vi "ziExample-Module-Impedance.vi"() -> ()   [LabVIEW 2009]
doc: "Control a Zurich instrument device via the LabOne Labview API. \nRequirements: Zurich Instruments MFLI+IA/ MFIA\nThis example shows how to use retrieve impedance data and utilize the sweeper.\n\n© Zurich Instruments AG, www.zhinst.com"
uses:
  <instrlib>/Zurich Instruments LabOne/Public/Modules/ziTypeModSweeperImpedanceWave.ctl
  <instrlib>/Zurich Instruments LabOne/Public/Modules/ziTypeModEnum.ctl
  <instrlib>/Zurich Instruments LabOne/Public/Configure/ziSetValueDoubleArray.vi
  <instrlib>/Zurich Instruments LabOne/Public/Modules/ziModSetValueDoubleArray.vi
  <instrlib>/Zurich Instruments LabOne/Public/Modules/ziModSetValueBinaryArray.vi
  <instrlib>/Zurich Instruments LabOne/Public/Modules/ziModGetSweeperData.vi
  <instrlib>/Zurich Instruments LabOne/Public/Data/ziGetEventImpSample.vi
  <instrlib>/Zurich Instruments LabOne/Public/Configure/ziSetValueDouble.vi
  <instrlib>/Zurich Instruments LabOne/Public/Configure/ziGetValueDouble.vi
  <instrlib>/Zurich Instruments LabOne/Zurich Instruments LabOne.lvlib
  <vilib>/gmath/NI_Gmath.lvlib
panel:
  out "Frequency":dbl
  in  "auto/inputrange":bool caption="Auto"
  in  "voltage/range":dbl=1.0 caption="Range Voltage"
  in  "current/range":dbl=0.001 caption="Range Current"
  in  "output/amplitude":dbl=0.1 caption="Test Signal (V)"
  in  "auto/output":bool caption="Auto"
  in  "model":u16(ring)=1 caption="Model" items=["Rp || Cp", "Rs + Cs", "Rs + Ls", "G B", "D Cs", "Q Cs", "D Ls", "Q Ls", "Rp || Lp", "D Cp"]
  out "?":dbl(graph)
  out "?":dbl(graph)
  in  "Sweep":bool
  in  "Step":dbl=100.0
  in  "stopfreq":dbl=100000.0 caption="Stop Freq"
  in  "startfreq":dbl=1000.0 caption="Start Freq"
  out "Flags":bool[][](array[boolean])
  out "ImpedanceSweeperData":T1 {"bandwidthMode" format="%f"; "flags" format="%f"; "sampleFormat" format="%f"; "sweepMode" format="%f"; "sampleCount" format="%f"; "timestamp" format="%f"}
  in  "stop":bool
  out "IA Parameter 2":dbl
  out "IA Parameter 1":dbl format="%#_6p"
  out "Error Out":errorcluster
  in  "Address":string="DEV"
  out "Selected Device":string
  in  "subscribepath":string="imps/0/sample" caption="Subscribe Path"
  out "Param1":cluster{"grid":dbl[], "r_avg":dbl[]}(graph)
  out "Param 0":cluster{"grid":dbl[], "r_avg":dbl[]}(graph)
  # "ziExample-IMPModul.vi\nRequirements: MFLI + IA / MFIA\nsee block diagram for VI description"
  # "Tested Devices:\n\n- MFLI"
  # "VALID_INTERNAL\nVALID_USER\nAUTORANGE_GATING\n\nOVERFLOW_VOLTAGE\nOVERFLOW_CURRENT\nUNDERFLOW_VOLTAGE\nUNDERFLOW_CURRENT\nFREQ_EXACT\nFREQ_INTERPOLATION\nFREQ_EXTRAPOLATION\n\nSUPPRESSION_PARAM0\nSUPPRESSION_PARAM1\nFREQLIMIT_RANGE_VOLTAGE\nFREQLIMIT_RANGE_Current\nSTRONGCOMPENSATION_PARAM0\nSTRONGCOMPENSATION_PARAM1\n\n\nBWC_BIT0\nBWC_BIT1\nBWC_BIT2\nBWC_BIT3\nOPEN_DETECTION"
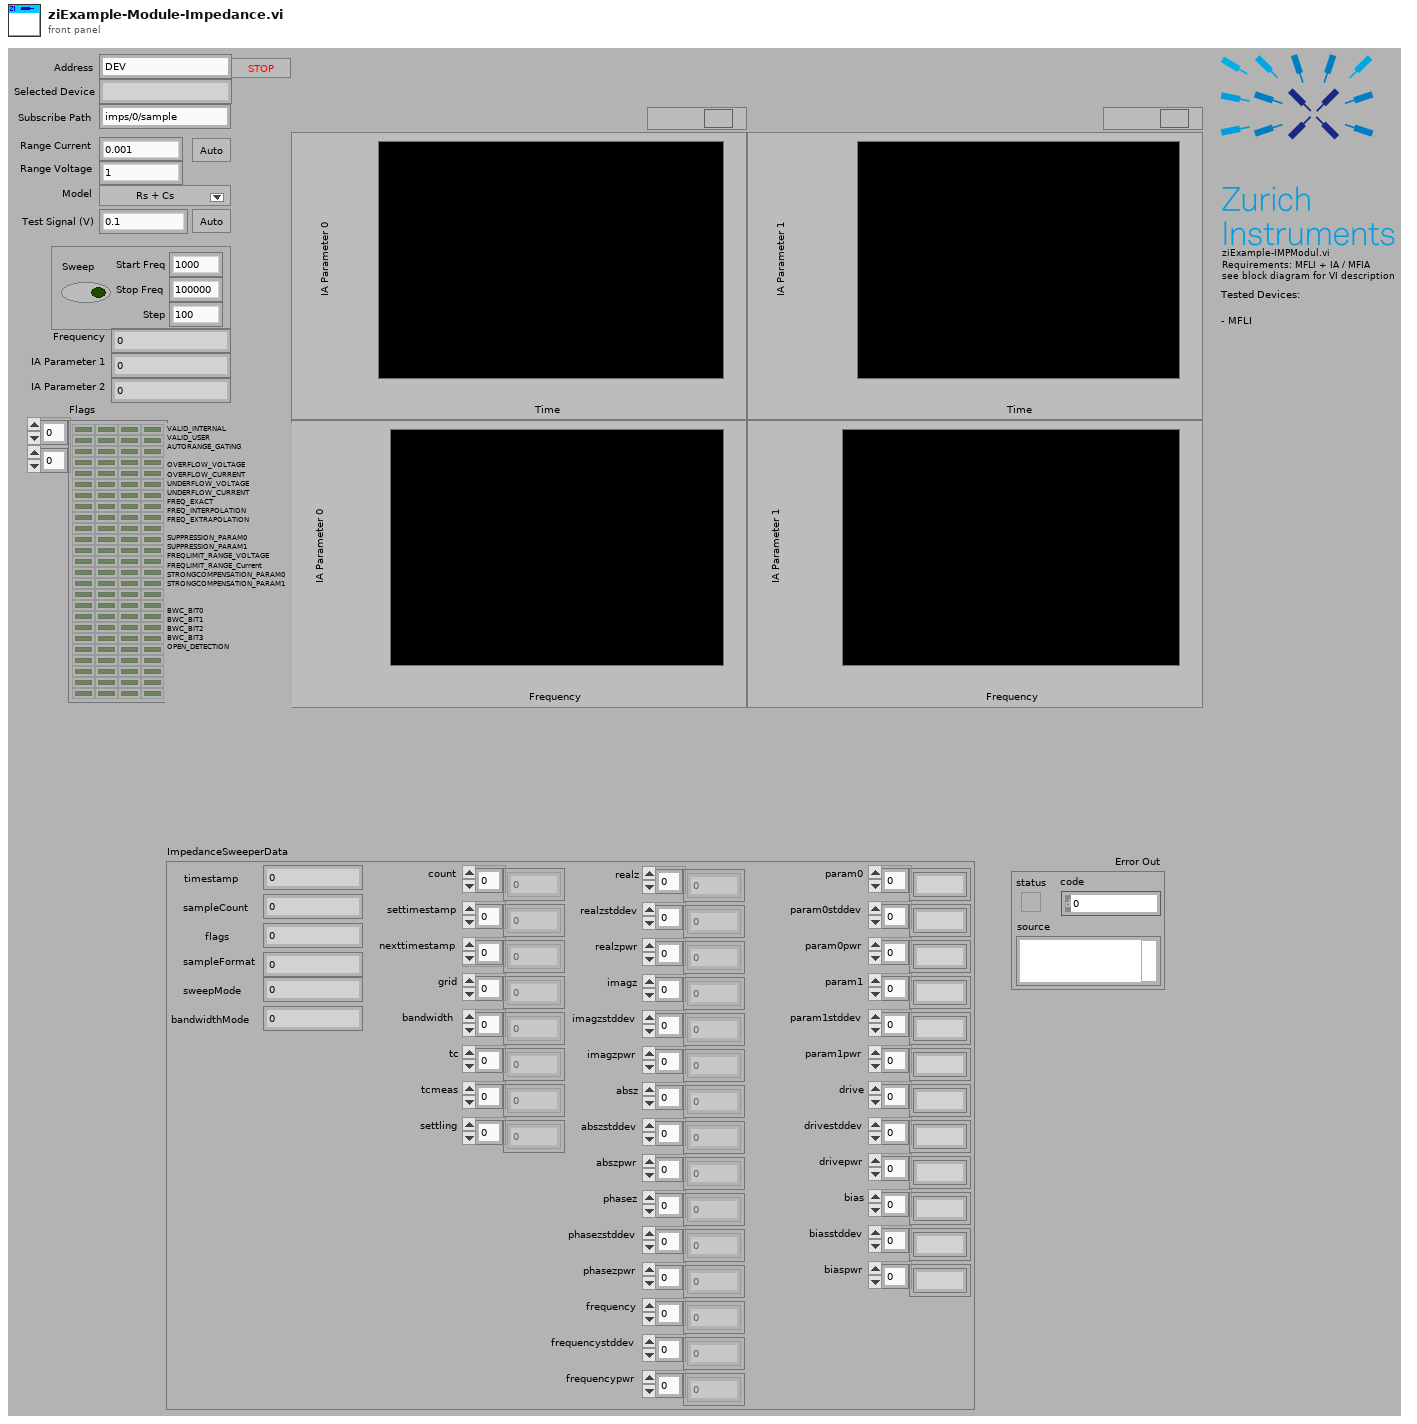
[diagram p1: front panel]
types:
  T1 = typedef "Zurich Instruments LabOne.lvlib/ziTypeModSweeperImpedanceWave.ctl" = cluster{"timestamp":u64, "sampleCount":u64, "flags":u8, "sampleFormat":u8, "sweepMode":u8, "bandwidthMode":u8, "count":u64[], "settimestamp":u64[], "nexttimestamp":u64[], "grid":dbl[], "bandwidth":dbl[], "tc":dbl[], "tcmeas":dbl[], "settling":dbl[], "realz":dbl[], "realzstddev":dbl[], "realzpwr":dbl[], "imagz":dbl[], "imagzstddev":dbl[], "imagzpwr":dbl[], "absz":dbl[], "abszstddev":dbl[], "abszpwr":dbl[], "phasez":dbl[], "phasezstddev":dbl[], "phasezpwr":dbl[], "frequency":dbl[], "frequencystddev":dbl[], "frequencypwr":dbl[], "param0":dbl[], "param0stddev":dbl[], "param0pwr":dbl[], "param1":dbl[], "param1stddev":dbl[], "param1pwr":dbl[], "drive":dbl[], "drivestddev":dbl[], "drivepwr":dbl[], "bias":dbl[], "biasstddev":dbl[], "biaspwr":dbl[]}
  T2 = typedef "Zurich Instruments LabOne.lvlib/ziTypeModEnum.ctl" = u16
  T3 = typedef "Zurich Instruments LabOne.lvlib/ziTypeHandle.ctl" = cluster{"handleValid":bool, "Conn":u64, "Path Prefix":string, "Handle":u64, "Connected":bool, "Clockbase(s)":dbl}
  T4 = typedef "Zurich Instruments LabOne.lvlib/ziTypeModHandle.ctl" = cluster{"handleValid":bool, "Conn":u64, "ModHandle":u64, "moduleID":string, "Path Prefix":string}
  T5 = typedef "Zurich Instruments LabOne.lvlib/ziTypeModResults.ctl" = cluster{"PathArray":string[], "ValueType":T6, "NoOfResults":u64, "ziGenericHeader":T7[]}
  T6 = typedef "Zurich Instruments LabOne.lvlib/ziTypePollType.ctl" = enum16{"NONE", "DOUBLE_DATA", "INTEGER_DATA", "DEMOD_SAMPLE", "SCOPE_WAVE_HF2", "AUXIN_SAMPLE", "DIO_SAMPLE", "BYTE_ARRAY", "PWA_WAVE", "9", "10", "11", "12", "13", "14", "15", "TREE_CHANGE_DEPRI", "17", "ERROR", "19", "20", "21", "22", "23", "24", "25", "26", "27", "28", "29", "30", "31", "DOUBLE_DATA_TS", "INTEGER_DATA_TS", "34", "SCOPE_WAVE", "SCOPE_WAVE_EX", "37", "BYTE_ARRAY_TS", "39", "40", "41", "42", "43", "44", "45", "CNT_DATA", "47", "TREE_CHANGE", "49", "50", "51", "52", "53", "54", "55", "56", "57", "58", "59", "60", "61", "62", "63", "SWEEPER_DATA", "SPECTRUM_DATA", "ADVISOR_DATA", "VECTOR_DATA", "IMP_DATA"}
  T7 = typedef "Zurich Instruments LabOne.lvlib/ziTypeModGenericHeader.ctl" = cluster{"HeaderType":enum8{"HEADER_TYPE_NONE", "HEADER_TYPE_SWTRIGGER", "HEADER_TYPE_SWEEPER"}, "SampleFormat":u8, "SystemTime":timestamp, "CreatedTimeStamp":u64, "ChangedTimeStamp":u64, "Flags":u32, "ChunkSizeBytes":u64, "Name":string, "Status":u32, "GroupIndex":u32, "Color":u32, "ActiveRow":u32, "TriggerNumber":u64, "GridRows":u32, "GridCols":u32, "GridMode":u32, "GridOperation":u32, "GridDirection":u32, "GridRepetitions":u32, "GridColDelta":dbl, "GridColOffset":dbl, "GridRowDelta":dbl, "GridRowOffset":dbl, "Bandwidth":dbl, "Center":dbl, "Nenbw":dbl}
  T8 = typedef "Zurich Instruments LabOne.lvlib/ziTypeImpedanceSample.ctl" = cluster{"Timestamps (ticks)":u64[], "Z (Ohm)":cdb[], "Freq (Hz)":dbl[], "Osc Phase (deg)":dbl[], "Flags":u32[], "Trigger":u32[], "Param0":dbl[], "Param1":dbl[], "Drive":dbl[], "Bias":dbl[]}
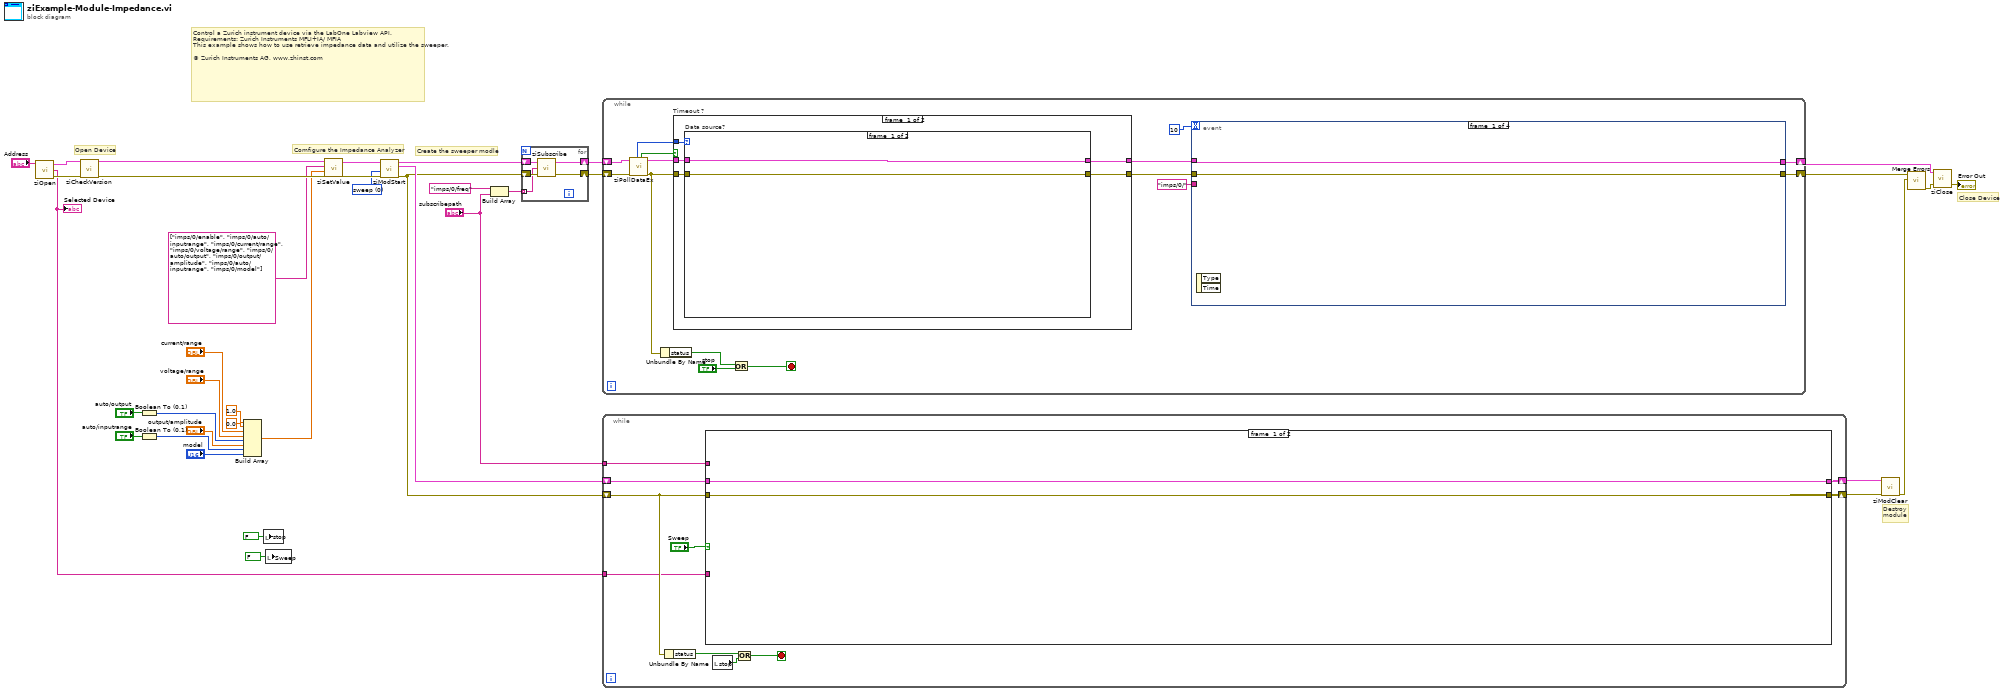
[diagram p0: block diagram]
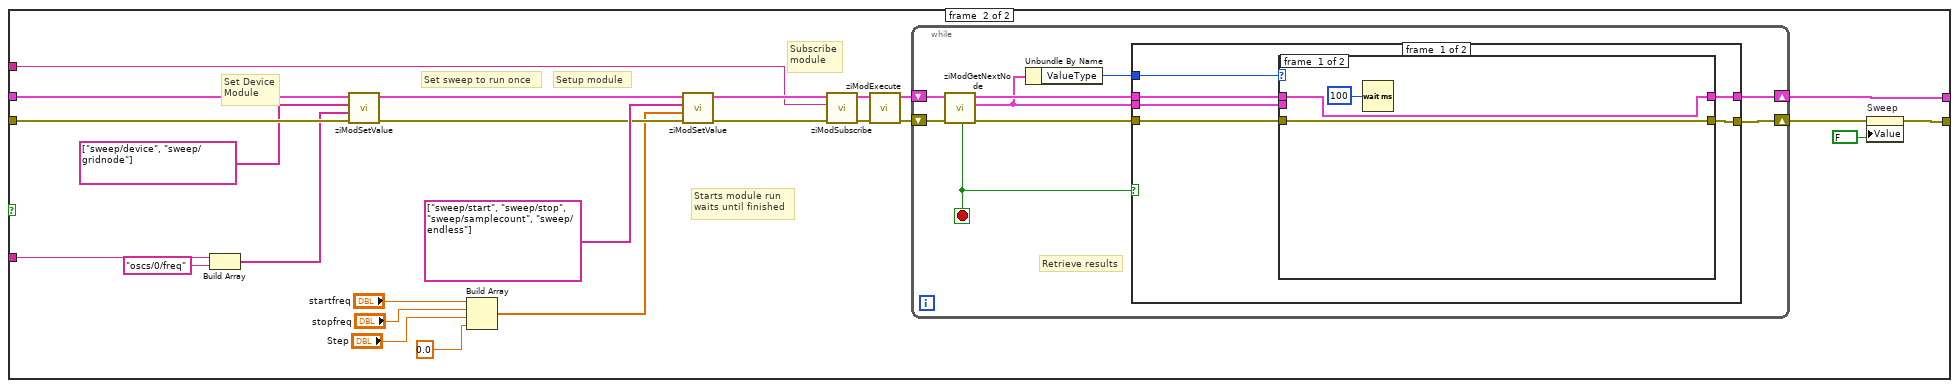
[diagram p2: hidden frame]
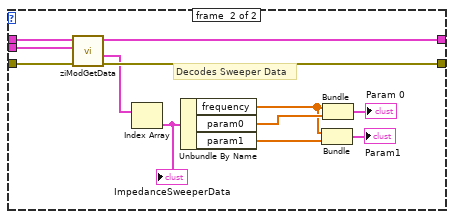
[diagram p3: hidden frame]
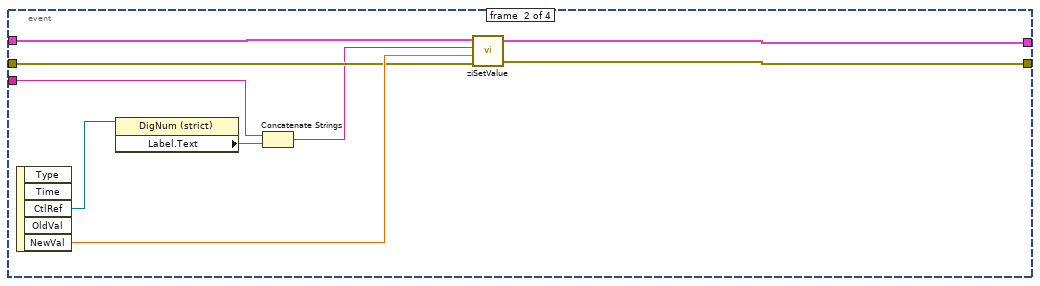
[diagram p5: hidden frame]
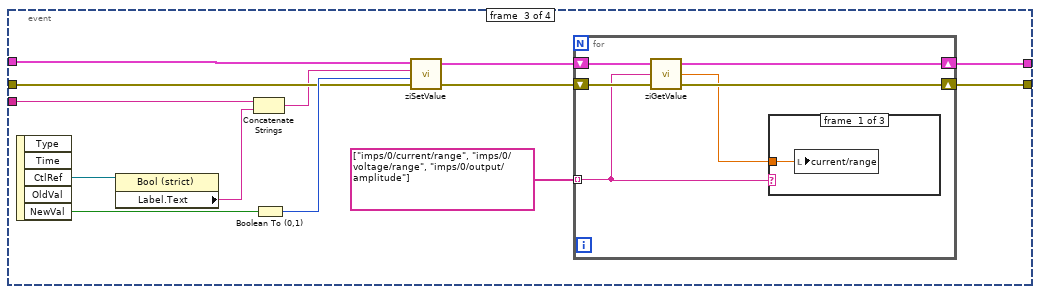
[diagram p6: hidden frame]
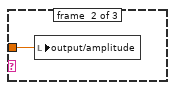
[diagram p7: hidden frame]
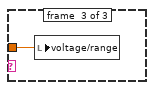
[diagram p8: hidden frame]
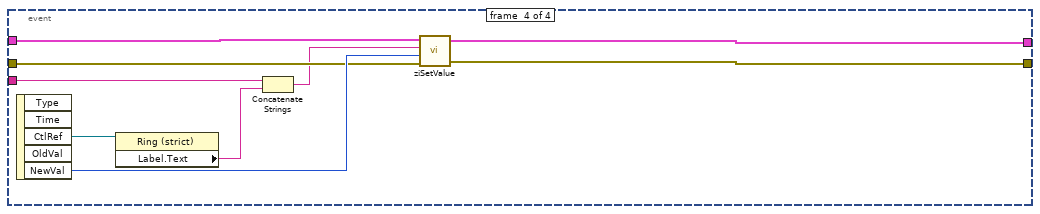
[diagram p9: hidden frame]
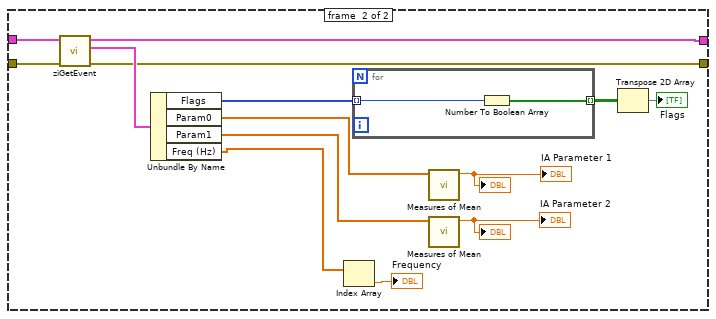
[diagram p10: hidden frame]
diagram:
  w21 = T2 0 items=["sweep", "scopeModule", "dataAcquisitionModule", "pidAdvisor", "awgModule", "impedanceModule", "multiDeviceSyncModule", "zoomFFT", "trigger", "deviceSettings", "record"] ("module Id")
  # "Comfigure the Impedance Analyzer"
  # "Destroy\nmodule"
  # "Control a Zurich instrument device via the LabOne Labview API. \nRequirements: Zurich Instruments MFLI+IA/ MFIA\nThis example shows how to use retrieve impedance data and utilize the sweeper.\n\n© Zurich Instruments AG, www.zhinst.com"
  # "Create the sweeper modle"
  # "Close Device"
  # "Open Device"
  n1 = call <instrlib>:"ziOpen.vi"("Address"="Address") -> ("Error Out"=w24:errorcluster, "Selected Device"=w3:string, "HandleOut"=w25:T3)  [unwired: 1 in, 2 out]
  "Selected Device" <- w3
  n2 = call <instrlib>:"ziCheckVersion.vi"("Handle In"=w25, "Error In"=w24) -> ("Handle Out"=w22:T3, "Error Out"=w23:errorcluster)  [unwired: 11 in, 1 out]
  n3 = Boolean To (0,1)(Boolean="auto/output") -> (0, 1=w13:i16)
  n4 = Boolean To (0,1)(Boolean="auto/inputrange") -> (0, 1=w14:i16)
  n5 = Build Array(1.0 ("element"), 0.0 ("element"), "current/range", "voltage/range", w13, "output/amplitude", w14, "model") -> (w9:dbl[])
  n6 = local write "stop"(FALSE ("stop")) -> ()
  n7 = local write "Sweep"(FALSE ("Sweep")) -> ()
  n8 = call-poly <instrlib>:"ziSetValue.vi"("Error In"=w23, "Values"=w9, "Paths"=string[] ["imps/0/enable", "imps/0/auto/inputrange", "imps/0/current/range", "imps/0/voltage/range", "imps/0/auto/output", "imps/0/output/amplitude", "imps/0/auto/inputrange", "imps/0/model"], "Handle In"=w22) -> ("Error Out"=w26:errorcluster, "Handle Out"=w27:T3)  [unwired: 1 in]
  n9 = call <instrlib>:"ziModStart.vi"("Error In"=w26, "module Id"=w21, "Handle In"=w27) -> ("Error Out"=w31:errorcluster, "ModHandle Out"=w38:T4, "Handle Out"=w34:T3)  [unwired: 6 in]
  n10 = Build Array("imps/0/freq", "subscribepath") -> (w6:string[])
  n11 = for {
    shift-right: [w42] -> w33
    shift-left: w34 -> [w43]
    shift-right: [w41] -> w32
    shift-left: w31 -> [w40]
    tunnel: w6 -> [w39] mode=indexing
    n12 = call <instrlib>:"ziSubscribe.vi"("error in"=w40, "Path ()"=w39, "Handle In"=w43) -> ("error out"=w41:errorcluster, "Handle Out"=w42:T3)  [unwired: 1 in]
  }
  n13 = while {
    shift-right: [w51] -> w36
    shift-left: w38 -> [w53]
    shift-right: [w52] -> w37
    shift-left: w31 -> [w50]
    tunnel: "subscribepath" -> [w45]
    tunnel: w3 -> [w44]
    stop <- w47 stop-if-true
    n14 = Unbundle By Name(w50) -> ("status"=w48:bool)
    n15 = case shown="True" "Sweep" {
      tunnel: w53 -> [w55 w80]
      tunnel: [w54 w79] -> w52
      tunnel: [w55 w78] -> w51
      tunnel: w50 -> [w54 w77]
      tunnel: w45 -> [_ w57]
      tunnel: w44 -> [_ w56]
      frame #0 {
      }
      frame #1 {
        # "Set Device\nModule"
        # "Starts module run\nwaits until finished"
        # "Set sweep to run once"
        # "Subscribe\nmodule"
        # "Setup module"
        n16 = Build Array(w56, "oscs/0/freq") -> (w64:string[])
        n17 = call-poly <instrlib>:"ziModSetValue.vi"("Error In"=w77, "Values"=w64, "Paths"=string[] ["sweep/device", "sweep/gridnode"], "ModHandle In"=w80) -> ("Error Out"=w70:errorcluster, "ModHandle Out"=w73:T4)  [unwired: 6 in]
        n18 = Build Array("startfreq", "stopfreq", "Step", 0.0 ("Value")) -> (w66:dbl[])
        n19 = call-poly <instrlib>:"ziModSetValue.vi"("Error In"=w70, "Values"=w66, "Paths"=string[] ["sweep/start", "sweep/stop", "sweep/samplecount", "sweep/endless"], "ModHandle In"=w73) -> ("Error Out"=w71:errorcluster, "ModHandle Out"=w72:T4)  [unwired: 6 in]
        n20 = call <instrlib>:"ziModSubscribe.vi"("Error In"=w71, "Path"=w57, "ModHandle In"=w72) -> ("Error Out"=w67:errorcluster, "ModHandle Out"=w68:T4)  [unwired: 6 in]
        n21 = call <instrlib>:"ziModExecute.vi"("Error In"=w67, "ziModHandle In"=w68) -> ("Error Out"=w75:errorcluster, "ziModHandle Out"=w76:T4)  [unwired: 7 in]
        n22 = while {
          shift-right: [w86] -> w78
          shift-left: w76 -> [w88]
          shift-right: [w85] -> w62
          shift-left: w75 -> [w89]
          stop <- w81 stop-if-true
          # "Retrieve results"
          n23 = call <instrlib>:"ziModGetNextNode.vi"("Error In"=w89, "ModHandle In"=w88) -> ("Error Out"=w82:errorcluster, "ModResults"=w84:T5, "ModHandle Out"=w87:T4, "NoData"=w81:bool)  [unwired: 6 in]
          n24 = Unbundle By Name(w84) -> ("ValueType"=w83:T6)
          n25 = case shown="False" w81 {
            tunnel: w87 -> [w95 w111]
            tunnel: [w94 w111] -> w86
            tunnel: [w93 w112] -> w85
            tunnel: w82 -> [w92 w112]
            tunnel: w84 -> [w91 _]
            tunnel: w83 -> [w90 _]
            frame #0 {
              n26 = case shown="\"SWEEPER_DATA\"" w90 {
                tunnel: w95 -> [w98 w109]
                tunnel: w91 -> [_ w110]
                tunnel: w92 -> [w97 w108]
                tunnel: [w97 w107] -> w93
                tunnel: [w98 w106] -> w94
                frame #0 {
                  n27 = Wait (ms)(milliseconds to wait=u32 100) -> ()  [unwired: 1 out]
                }
                frame #1 {
                  # "Decodes Sweeper Data"
                  n28 = call-poly <instrlib>:"ziModGetData.vi"("Error In"=w108, "ModResults"=w110, "ModHandle In"=w109) -> ("Error Out"=w107:errorcluster, "SweeperImpedanceWaveArray"=w100:T1[], "ModHandle Out"=w106:T4)  [unwired: 4 in, 2 out]
                  n29 = Index Array(array=w100) -> (element=w99:T1)  [unwired: 1 in]
                  "ImpedanceSweeperData" <- w99
                  n30 = Unbundle By Name(w99) -> ("frequency"=w101:dbl[], "param0"=w105:dbl[], "param1"=w102:dbl[])
                  n31 = Bundle("frequency"=w101, "param1"=w102) -> (→"Param1":cluster{"frequency":dbl[], "param1":dbl[]})  [unwired: 1 in]
                  n32 = Bundle("frequency"=w101, "param0"=w105) -> (→"Param 0":cluster{"frequency":dbl[], "param0":dbl[]})  [unwired: 1 in]
                }
              }
            }
            frame #1 {
            }
          }
        }
        n33 = property on="Sweep" class="Bool (strict)"(error in=w62, "Value"=FALSE ("Sweep")) -> (error out=w79:errorcluster)  [unwired: 1 in, 1 out]
      }
    }
    n34 = local read "stop"() -> (w49:bool)
    n35 = Or(x=w48, y=w49) -> (x .or. y?=w47:bool)
  }
  n36 = while {
    shift-right: [w116] -> w29
    shift-left: w32 -> [w119]
    shift-right: [w117] -> w35
    shift-left: w33 -> [w120]
    stop <- w121 stop-if-true
    n37 = call <instrlib>:"ziPollDataEx.vi"("error in"=w119, "Handle In"=w120) -> ("error out"=w124:errorcluster, "Handle Out"=w126:T3, "Timed Out"=w127:bool, "ziValueType"=w125:T6)  [unwired: 2 in, 4 out]
    n38 = Unbundle By Name(w124) -> ("status"=w122:bool)
    n39 = case "Timeout ?" shown="False" w127 {
      tunnel: w126 -> [w174 w194]
      tunnel: [w173 w194] -> w118
      tunnel: w124 -> [w172 w193]
      tunnel: [w170 w193] -> w115
      tunnel: w125 -> [w171 _]
      frame #0 {
        n40 = case "Data source?" shown="\"IMP_DATA\"" w171 {
          tunnel: w174 -> [w176 w190]
          tunnel: [w176 w186] -> w173
          tunnel: w172 -> [w175 w188]
          tunnel: [w175 w187] -> w170
          frame #0 {
          }
          frame #1 {
            n41 = call-poly <instrlib>:"ziGetEvent.vi"("Error In"=w188, "Handle In"=w190) -> ("Error Out"=w187:errorcluster, "Imp Sample Out"=w189:T8, "Handle Out"=w186:T3)  [unwired: 7 in]
            n42 = Unbundle By Name(w189) -> ("Flags"=w185:u32[], "Param0"=w182:dbl[], "Param1"=w181:dbl[], "Freq (Hz)"=w178:dbl[])
            n43 = Index Array(array=w178) -> (element=→"Frequency":dbl)  [unwired: 1 in]
            n44 = for {
              tunnel: w185 -> [w192] mode=indexing
              tunnel: [w191] -> w184 mode=indexing
              n45 = Number To Boolean Array(number=w192) -> (Boolean array=w191:bool[])
            }
            n46 = call <vilib>:"Measures of Mean.vi"("x array"=w182) -> ("mean value"=→"IA Parameter 1" →"?":dbl)  [unwired: 9 in, 1 out]
            n47 = call <vilib>:"Measures of Mean.vi"("x array"=w181) -> ("mean value"=→"IA Parameter 2" →"?":dbl)  [unwired: 9 in, 1 out]
            n48 = Transpose 2D Array(2D array=w184) -> (transposed array=→"Flags":bool[][])
          }
        }
      }
      frame #1 {
        # "Timeout, no action."
      }
    }
    n49 = Or(x=w122, y="stop") -> (x .or. y?=w121:bool)
    n50 = event shown="[1] \"voltage/range\", \"current/range\", \"output/amplitude\": Value Change" {
      selector: _ -> [_ _ _ _]
      dyn-events: _ -> [_ _ _ _]
      timeout: 10 -> [_ _ _ _]
      tunnel: w118 -> [w129 w136 w149 w164]
      tunnel: [w129 w135 w141 w167] -> w117
      tunnel: [w128 w134 w140 w166] -> w116
      tunnel: w115 -> [w128 w133 w148 w165]
      tunnel: "imps/0/" -> [_ w132 w145 w161]
      event #0 {
        n51 = event-data() -> ()  [unwired: 1 in, 2 out]
      }
      event #1 {
        n52 = event-data() -> ("CtlRef"=w138:refnum<vi>, "NewVal"=w137:dbl)  [unwired: 1 in, 3 out]
        n53 = property class="DigNum (strict)"(reference=w138) -> ("Label.Text"=w131:string)  [unwired: 1 in, 2 out]
        n54 = Concatenate Strings(w132, w131) -> (w130:string)
        n55 = call-poly <instrlib>:"ziSetValue.vi"("Error In"=w133, "Value"=w137, "Path"=w130, "Handle In"=w136) -> ("Error Out"=w134:errorcluster, "Handle Out"=w135:T3)  [unwired: 1 in]
      }
      event #2 {
        n56 = event-data() -> ("CtlRef"=w151:refnum<vi>, "NewVal"=w144:bool)  [unwired: 1 in, 3 out]
        n57 = property class="Bool (strict)"(reference=w151) -> ("Label.Text"=w146:string)  [unwired: 1 in, 2 out]
        n58 = Concatenate Strings(w145, w146) -> (w147:string)
        n59 = Boolean To (0,1)(Boolean=w144) -> (0, 1=w150:i16)
        n60 = call-poly <instrlib>:"ziSetValue.vi"("Error In"=w148, "Value"=w150, "Path"=w147, "Handle In"=w149) -> ("Error Out"=w142:errorcluster, "Handle Out"=w143:T3)  [unwired: 1 in]
        n61 = for {
          tunnel: string[] ["imps/0/current/range", "imps/0/voltage/range", "imps/0/output/amplitude"] -> [w155] mode=indexing
          shift-right: [w153] -> w140
          shift-left: w142 -> [w156]
          shift-right: [w154] -> w141
          shift-left: w143 -> [w157]
          n62 = call-poly <instrlib>:"ziGetValue.vi"("error in"=w156, "Path"=w155, "Handle in"=w157) -> ("error out"=w153:errorcluster, "Value"=w152:dbl, "Handle out"=w154:T3)
          n63 = case shown="\"imps/0/current/range\", Default" w155 {
            tunnel: w152 -> [w158 w159 w160]
            frame #0 {
              n64 = local write "current/range"(w158) -> ()
            }
            frame #1 {
              n65 = local write "output/amplitude"(w159) -> ()
            }
            frame #2 {
              n66 = local write "voltage/range"(w160) -> ()
            }
          }
        }
      }
      event #3 {
        n67 = event-data() -> ("CtlRef"=w169:refnum<vi>, "NewVal"=w168:u16)  [unwired: 1 in, 3 out]
        n68 = property class="Ring (strict)"(reference=w169) -> ("Label.Text"=w162:string)  [unwired: 1 in, 2 out]
        n69 = Concatenate Strings(w161, w162) -> (w163:string)
        n70 = call-poly <instrlib>:"ziSetValue.vi"("Error In"=w165, "Value"=w168, "Path"=w163, "Handle In"=w164) -> ("Error Out"=w166:errorcluster, "Handle Out"=w167:T3)  [unwired: 1 in]
      }
    }
  }
  n71 = call <instrlib>:"ziModClear.vi"("Error In"=w37, "ziModHandle In"=w36) -> ("Error Out"=w30:errorcluster)  [unwired: 7 in, 1 out]
  n72 = call <vilib>:"Merge Errors.vi"("error in 2 (no error)"=w30, "error in 1 (no error)"=w29) -> ("error out"=w28:errorcluster)  [unwired: 5 in]
  n73 = call <instrlib>:"ziClose.vi"("Error In"=w28, "Handle In"=w35) -> ("Error Out"=→"Error Out":errorcluster)  [unwired: 2 in, 1 out]
